vi "sub_PwrPak7_parsing.vi"(11 "gps recevied data":string) -> (3 "utm-1":cluster{"XN":dbl, "YE":dbl}={"XN"=530126.7583503594, "YE"=175270.68061157822} {"XN" format="%.2f"; "YE" format="%.2f"})   [LabVIEW 2019]
uses:
  Ctrl/gps-databuf.ctl
  Ctrl/log_buffq.ctl
panel:
  out "mode chk":bool
  out "head chk":bool
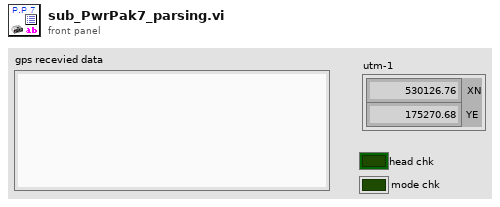
[diagram p1: front panel]
types:
  T1 = typedef "gps-databuf.ctl" = enum16{"read", "write"}
  T2 = typedef "log_buffq.ctl" = enum16{"create", "write", "read", "close"}
  T3 = cluster{"rawdata":string, "GPS Data":cluster{"Latitude":cluster{"Valid?":bool, "Latitude (Deg)":dbl}, "Longitude":cluster{"Valid?":bool, "Longitude (Deg)":dbl}, "Height":cluster{"Valid?":bool, "Height (m)":dbl}, "Undulation":cluster{"Valid?":bool, "Undulation(m)":dbl}, "North Vel":cluster{"Valid?":bool, "North Vel (m/s)":dbl}, "East Vel":cluster{"Valid?":bool, "East Vel (m/s)":dbl}, "Up Vel":cluster{"Valid?":bool, "Up Vel (m/s)":dbl}, "Roll":cluster{"Valid?":bool, "Roll (degrees)":dbl}, "Pitch":cluster{"Valid?":bool, "Pitch (degrees)":dbl}, "Azimuth":cluster{"Valid?":bool, "Azimuth (degrees)":dbl}, "Lat deviation":cluster{"Valid?":bool, "Lat deviation (m)":dbl}, "Long deviation":cluster{"Valid?":bool, "Long deviation (m)":dbl}, "Height deviation":cluster{"Valid?":bool, "Height deviation (m)":dbl}, "North vel deviation":cluster{"Valid?":bool, "North vel deviation (m/s)":dbl}, "East vel deviation":cluster{"Valid?":bool, "East vel deviation (m/s)":dbl}, "Up vel deviation":cluster{"Valid?":bool, "Up vel deviation (m/s)":dbl}, "Roll deviation":cluster{"Valid?":bool, "Roll deviation (degrees)":dbl}, "Pitch deviation":cluster{"Valid?":bool, "Pitch deviation (degrees)":dbl}, "Azimuth deviation":cluster{"Valid?":bool, "Azimuth deviation (degrees)":dbl}, "Ext sol status":cluster{"Valid?":bool, "Ext sol status":dbl}}, "Heading":dbl, "utm-1":cluster{"XN":dbl, "YE":dbl}}
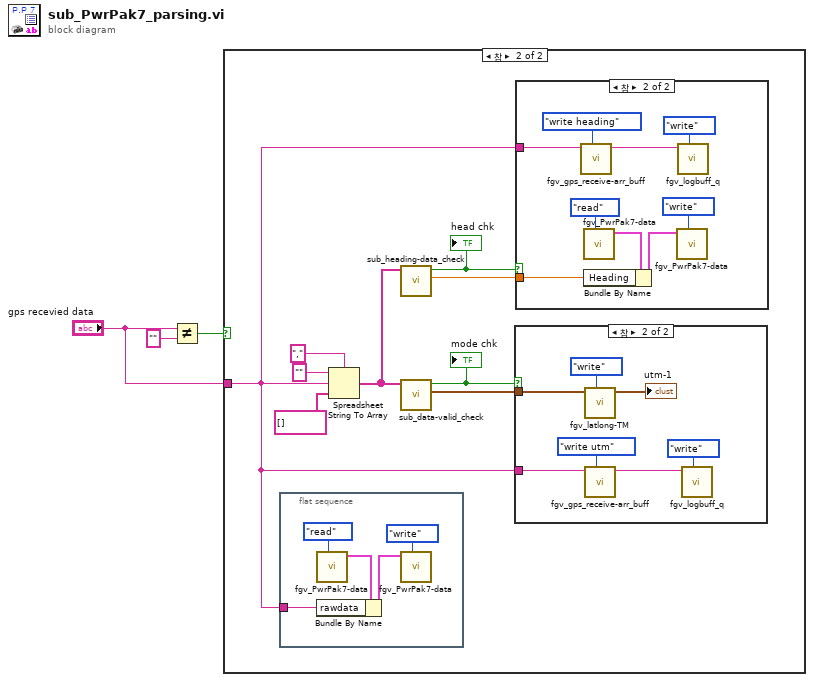
[diagram p0: block diagram]
diagram:
  n1 = Not Equal?(x="gps recevied data", y="") -> (x != y?=w1:bool)
  n2 = case shown="참" w1 {
    tunnel: "gps recevied data" -> [_ w4]
    frame False {
    }
    frame True {
      n3 = flat-sequence {
        tunnel: w4 -> [w13]
        frame #0 {
          n4 = call "fgv_PwrPak7-data.vi"("cmd"=gps-databuf."read") -> ("data cluster out"=w17:T3)  [unwired: 9 in, 1 out]
          n5 = Bundle By Name(cluster=w17, "rawdata"=w13) -> (w16:T3)
          n6 = call "fgv_PwrPak7-data.vi"("cmd"=gps-databuf."write", "data cluster in"=w16) -> ()  [unwired: 8 in, 2 out]
        }
      }
      n7 = Spreadsheet String To Array(delimiter (Tab)="," ("구분 문자 (탭)"), format string="" ("포맷 문자열"), spreadsheet string=w4, array type (2D Dbl)=string[] []) -> (array=w10:string[])
      n8 = call "sub_heading-data_check.vi"("gps received data-arr"=w10) -> ("heading"=w11:dbl, "heading_check"=w12:bool)  [unwired: 8 in, 1 out]
      "head chk" <- w12
      n9 = call "sub_data-valid_check.vi"("gps receive parsing array"=w10) -> ("utm-1"=w8:cluster{dbl, dbl}, "mode check"=w9:bool)  [unwired: 8 in, 1 out]
      "mode chk" <- w9
      n10 = case shown="참" w9 {
        tunnel: w8 -> [_ w32]
        tunnel: w4 -> [_ w28]
        frame False {
        }
        frame True {
          n11 = call "fgv_latlong-TM.vi"("cmd"=enum16{"write", "read"}."write", "latlong"=w32) -> ("latlong out"=→"utm-1":cluster{dbl, dbl})  [unwired: 8 in, 1 out]
          n12 = call "fgv_gps_receive-arr_buff.vi"("cmd"=enum16{"read", "write utm", "write heading"}."write utm", "gps receive str"=w28) -> ("gps log out"=w27:string)  [unwired: 8 in, 1 out]
          n13 = call "fgv_logbuff_q.vi"("cmd"=log_buffq."write", "data"=w27) -> ()  [unwired: 8 in, 2 out]
        }
      }
      n14 = case shown="참" w12 {
        tunnel: w11 -> [_ w22]
        tunnel: w4 -> [_ w19]
        frame False {
        }
        frame True {
          n15 = call "fgv_gps_receive-arr_buff.vi"("cmd"=enum16{"read", "write utm", "write heading"}."write heading", "gps receive str"=w19) -> ("gps log out"=w18:string)  [unwired: 8 in, 1 out]
          n16 = call "fgv_PwrPak7-data.vi"("cmd"=gps-databuf."read") -> ("data cluster out"=w24:T3)  [unwired: 9 in, 1 out]
          n17 = Bundle By Name(cluster=w24, "Heading"=w22) -> (w23:T3)
          n18 = call "fgv_PwrPak7-data.vi"("cmd"=gps-databuf."write", "data cluster in"=w23) -> ()  [unwired: 8 in, 2 out]
          n19 = call "fgv_logbuff_q.vi"("cmd"=log_buffq."write", "data"=w18) -> ()  [unwired: 8 in, 2 out]
        }
      }
    }
  }
